vi "SG_5GsetupEVM.vi"(5 "SG_WFM_FILE":path=path "D:/_Project/_Code/LabVIEW/CLC_Gen4/L2_Cali/CLC_Gen4_L2_InPhaseCal_Power/Config/wav/re11be_waveform/QC_WIFI_11BE_EHT320-1_LDPC_MCSB.wfm", 7 "max_dBm":i32, 8 "error in":errorcluster, 11 "VISA in":refnum<visa-resource-name>) -> (0 "error out":errorcluster, 2 "SG_Resp":string, 3 "VISA out":refnum<visa-resource-name>)   [LabVIEW 2023, in "Keysight.lvlib"]
uses:
  Keysight.lvlib
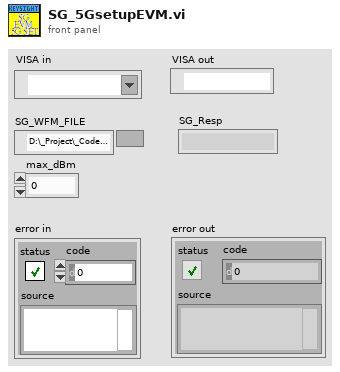
[diagram p1: front panel]
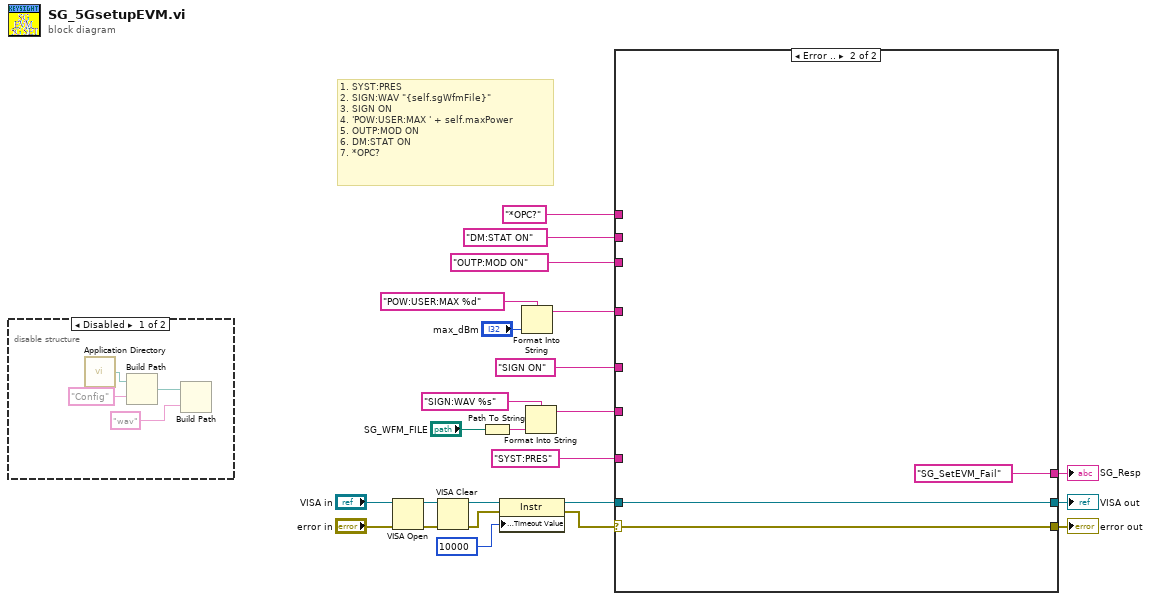
[diagram p0: block diagram]
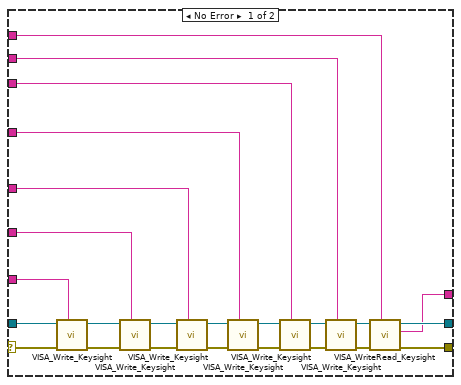
[diagram p3: hidden frame]
diagram:
  # "1. SYST:PRES\n2. SIGN:WAV \"{self.sgWfmFile}\"\n3. SIGN ON\n4. 'POW:USER:MAX ' + self.maxPower\n5. OUTP:MOD ON\n6. DM:STAT ON\n7. *OPC?"
  n1 = disable-structure shown="Disabled" {
    frame Disabled {
      n2 = call <vilib>:"Application Directory.vi"() -> ("Application Directory"=w27:path)
      n3 = Build Path(base path=w27, name or relative path="Config") -> (appended path=w26:path)
      n4 = Build Path(base path=w26, name or relative path="wav") -> ()  [unwired: 1 out]
    }
    frame Enabled {
    }
  }
  n5 = VISA Open(error in (no error)="error in", VISA resource name="VISA in") -> (VISA resource name=w5:refnum<visa-resource-name>, error out=w6:errorcluster)  [unwired: 3 in]
  n6 = VISA Clear(VISA resource name=w5, error in (no error)=w6) -> (VISA resource name out=w8:refnum<visa-resource-name>, error out=w7:errorcluster)
  n7 = Path To String(path="SG_WFM_FILE") -> (string=w21:string)
  n8 = property on="Property Node" class="Instr"(reference=w8, error in=w7, "General Settings:Timeout Value"=u32 10000) -> (reference out=w1:refnum<visa-resource-name>, error out=w2:errorcluster)
  n9 = Format Into String(format string="POW:USER:MAX %d", "max_dBm") -> (resulting string=w16:string)  [unwired: 2 in, 1 out]
  n10 = Format Into String(format string="SIGN:WAV %s", w21) -> (resulting string=w20:string)  [unwired: 2 in, 1 out]
  n11 = case shown="Error .." w2 {
    selector: w2 -> [w52 w54]
    tunnel: w1 -> [w51 w55]
    tunnel: "SYST:PRES" ("write buffer") -> [w50 _]
    tunnel: w20 -> [w47 _]
    tunnel: "SIGN ON" ("write buffer") -> [w44 _]
    tunnel: w16 -> [w41 _]
    tunnel: "OUTP:MOD ON" ("write buffer") -> [w38 _]
    tunnel: "DM:STAT ON" ("write buffer") -> [w33 _]
    tunnel: "*OPC?" ("write buffer") -> [w32 _]
    tunnel: [w31 w54] -> w10
    tunnel: [w30 w55] -> w11
    tunnel: [w29 "SG_SetEVM_Fail" ("Response")] -> w12
    frame No Error {
      n12 = call "VISA_Write_Keysight.vi"("VISA CMD"=w50, "error in"=w52, "VISA in"=w51) -> ("error out"=w49:errorcluster, "VISA out"=w48:refnum<visa-resource-name>)  [unwired: 7 in]
      n13 = call "VISA_Write_Keysight.vi"("VISA CMD"=w47, "error in"=w49, "VISA in"=w48) -> ("error out"=w46:errorcluster, "VISA out"=w45:refnum<visa-resource-name>)  [unwired: 7 in]
      n14 = call "VISA_Write_Keysight.vi"("VISA CMD"=w44, "error in"=w46, "VISA in"=w45) -> ("error out"=w43:errorcluster, "VISA out"=w42:refnum<visa-resource-name>)  [unwired: 7 in]
      n15 = call "VISA_Write_Keysight.vi"("VISA CMD"=w41, "error in"=w43, "VISA in"=w42) -> ("error out"=w40:errorcluster, "VISA out"=w39:refnum<visa-resource-name>)  [unwired: 7 in]
      n16 = call "VISA_Write_Keysight.vi"("VISA CMD"=w38, "error in"=w40, "VISA in"=w39) -> ("error out"=w37:errorcluster, "VISA out"=w36:refnum<visa-resource-name>)  [unwired: 7 in]
      n17 = call "VISA_Write_Keysight.vi"("VISA CMD"=w33, "error in"=w37, "VISA in"=w36) -> ("error out"=w35:errorcluster, "VISA out"=w34:refnum<visa-resource-name>)  [unwired: 7 in]
      n18 = call "VISA_WriteRead_Keysight.vi"("VISA_CMD"=w32, "error in"=w35, "VISA in"=w34) -> ("error out"=w31:errorcluster, "Response"=w29:string, "VISA out"=w30:refnum<visa-resource-name>)  [unwired: 6 in]
    }
    frame Error {
    }
  }
  "SG_Resp" <- w12
  "VISA out" <- w11
  "error out" <- w10
